vi "onComputeIntervals.vi"(8 "error in (no error)":errorcluster, 9 "Cron Interval":T1, 10 "Expression":string, 11 "Cron in":refnum<class "Cron.lvclass">) -> (0 "error out":errorcluster, 2 "Interval Parameters":T2, 3 "Cron out":refnum<class "Cron.lvclass">)   [LabVIEW 2013, in "openCron.lvlib" / "Cron.lvclass"]
uses:
  Cron.lvclass
  Cron Interval -- cluster.ctl
  Cron Interval -- enum.ctl
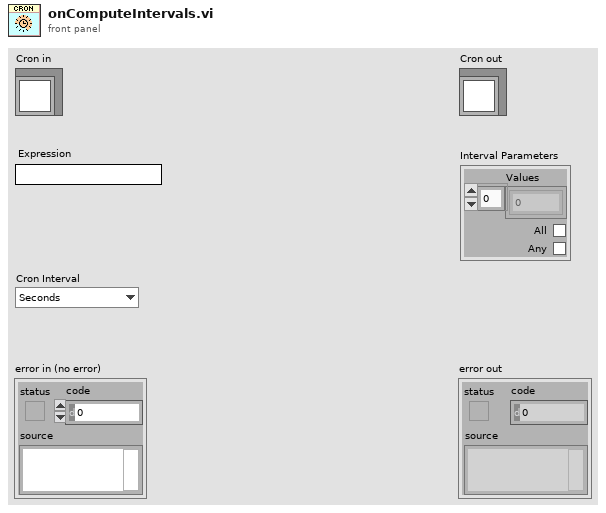
[diagram p1: front panel]
types:
  T1 = typedef "openCron.lvlib/Cron.lvclass/Cron Interval -- enum.ctl" = enum16{"Seconds", "Minutes", "Hours", "Day of Month", "Month", "Day of Week", "Year"}
  T2 = typedef "openCron.lvlib/Cron.lvclass/Cron Interval -- cluster.ctl" = cluster{"Values":i32[], "All":bool, "Any":bool}
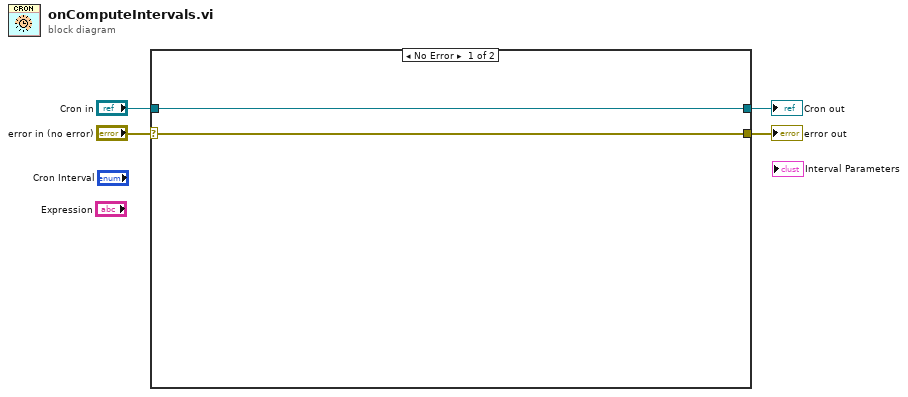
[diagram p0: block diagram]
diagram:
  n1 = case shown="No Error" "error in (no error)" {
    selector: "error in (no error)" -> [w5 w8]
    tunnel: [w5 w8] -> w3
    tunnel: [w6 w7] -> w1
    tunnel: "Cron in" -> [w6 w7]
    frame No Error {
    }
    frame Error {
    }
  }
  "error out" <- w3
  "Cron out" <- w1
